vi "RX OOB Test Cases.vi"() -> (0 "error out":errorcluster, 2 "status":string, 3 "pass":bool)   [LabVIEW 2021]
uses:
  CIFUtilities/CIFOutOfBand/CIFOutOfBand.lvclass/CIFOutOfBand.ctl
  OOB_Rx/Typedef/OOB Core Commands.ctl
  OOB_Rx/Private/Command Settings.vi
  CIFUtilities/CIFOutOfBand/Accessors/Write Local OOB Data.vi
  CIFUtilities/CIFOutOfBand/Write OOB DVR.vi
  CIFUtilities/CIFOutOfBand/Utilities/Command to Bitwise Command.vi
  CIFUtilities/CIFOutOfBand/Read OOB DVR.vi
  OOB_Rx/Private/Read Payload.vi
  OOB_Rx/CIFCoreOOB_Rx.lvclass
  D:/dev/CIF-LVCore/src/CIFUtilities/CIFOutOfBand/CIFOutOfBand.lvclass
  CIFUtilities/CIFOutOfBand/Init OOB.vi
  <vilib>/addons/_JKI.lib/Serialization/JSON/Library/Unflatten From JSON String.vi
  <vilib>/addons/_JKI.lib/Serialization/JSON/JKI JSON Serialization.lvlib
  CIFUtilities/CIFOutOfBand/CIFOutOfBand.lvclass
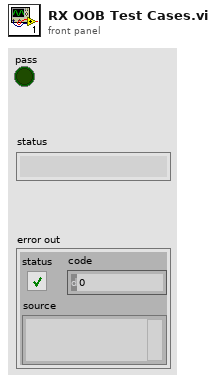
[diagram p1: front panel]
types:
  T1 = cluster{"Numeric":dbl, "Array":cluster{"Numeric":dbl, "String":string, "Boolean":bool}[], "string":string, "Null array":u8[]}
  T2 = typedef "CIFCoreOOB_Rx.lvclass/OOB Core Commands.ctl" = enum8{"Start", "StartFTE", "Pause", "Stop", "RefreshStats", "UpdateConfig"}
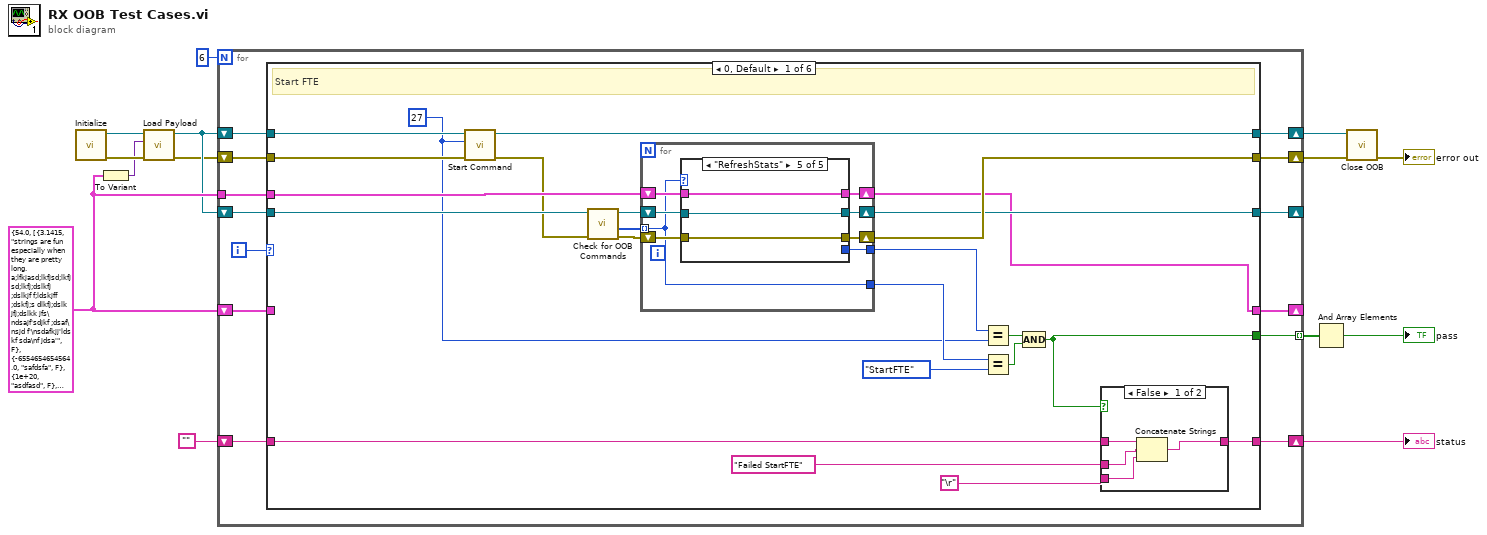
[diagram p0: block diagram]
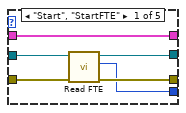
[diagram p2: hidden frame]
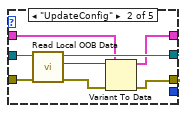
[diagram p3: hidden frame]
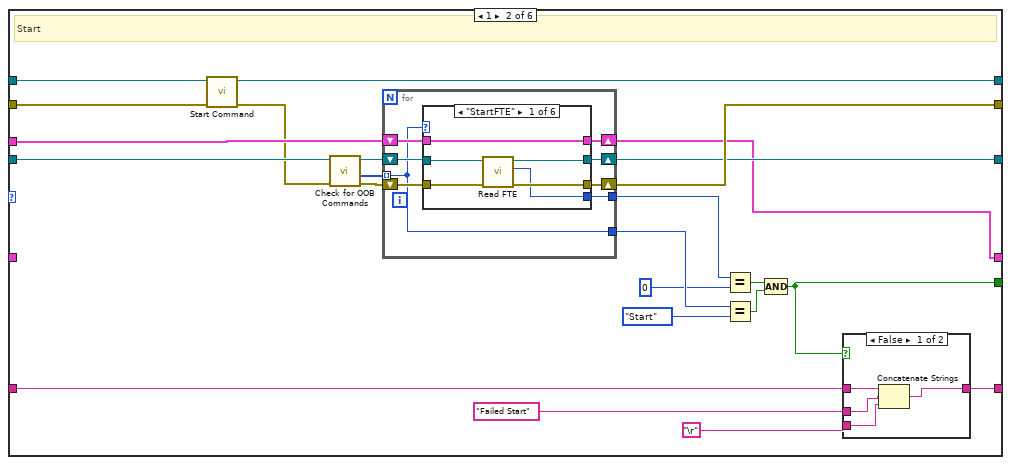
[diagram p7: hidden frame]
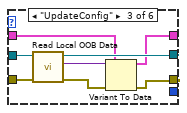
[diagram p9: hidden frame]
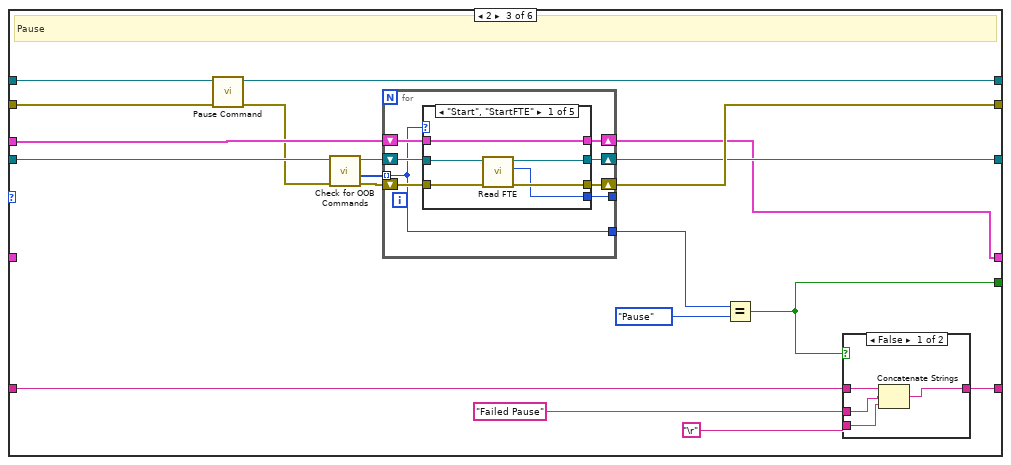
[diagram p14: hidden frame]
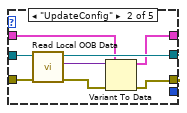
[diagram p15: hidden frame]
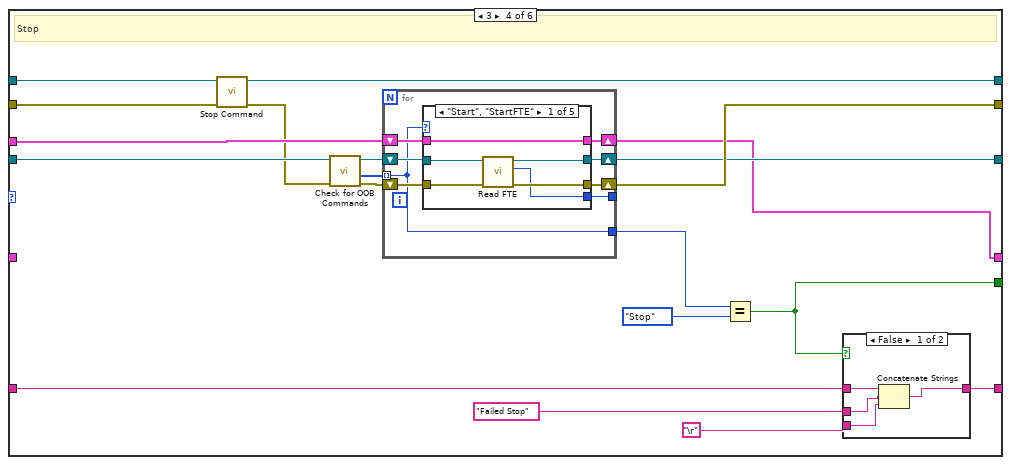
[diagram p20: hidden frame]
diagram:
  w14 = T1 {"Numeric"=54.0, "Array"=[{"Numeric"=3.1415, "String"="strings are fun especially when they are pretty long. a;lfkjasd;lkfjsd;lkfjsd;lkfj;dslkfj ;dslkjf f;ldskjff ;dskfj;s dlkfj;dslk jfj;dslkk jfs\ndsajf'sdjkf ;dsaf\nsjd f'\nsdafkjj'lds kf sda\nf jdsa'", "Boolean"=FALSE}, {"Numeric"=-6554654654564.0, "String"="safdsfa", "Boolean"=FALSE}, {"Numeric"=1e+20, "String"="asdfasd", "Boolean"=FALSE}, {"Numeric"=2.0, "String"="afd", "Boolean"=TRUE}, {"Numeric"=12.34, "String"="data", "Boolean"=FALSE}], "string"="strings", "Null array"=[0]} ("Test Config")
  n1 = call "Initialize.vi"() -> ("error out"=w7:errorcluster, "CoreOOB_Rx out"=w6:refnum<class "CIFCoreOOB_Rx.lvclass">)  [unwired: 10 in]
  n2 = To Variant(anything=w14) -> (Variant=w3:variant)
  n3 = call "Load Payload.vi"("error in (no error)"=w7, "Configuration Payload"=w3, "CoreOOB_Rx in"=w6) -> ("error out"=w4:errorcluster, "CoreOOB_Rx out"=w5:refnum<class "CIFCoreOOB_Rx.lvclass">)  [unwired: 7 in]
  n4 = for {
    N: 6 -> [_]
    tunnel: [w27] -> w11 mode=indexing
    tunnel: w14 -> [w25]
    shift-right: [w23] -> w12
    shift-left: w4 -> [w26]
    shift-right: [w21] -> w13
    shift-left: w5 -> [w24]
    shift-right: [w19] -> _
    shift-left: w5 -> [w20]
    shift-right: [w18] -> _
    shift-left: w14 -> [w17]
    shift-right: [w15] -> w8
    shift-left: "" -> [w16]
    i -> [w22]
    n5 = case shown="0, Default" w22 {
      tunnel: [w32 w91 w149 w208 w263 w325] -> w27
      tunnel: w26 -> [w41 w100 w152 w206 w261 w320]
      tunnel: w25 -> [w50 w109 w167 w222 w277 w318]
      tunnel: w24 -> [w42 w101 w153 w207 w262 w322]
      tunnel: [w49 w108 w166 w221 w276 w337] -> w23
      tunnel: [w40 w99 w150 w204 w259 w321] -> w21
      tunnel: w20 -> [w39 w98 w159 w214 w269 w331]
      tunnel: [w48 w107 w165 w220 w275 w336] -> w19
      tunnel: [w47 w106 w164 w219 w274 w314] -> w18
      tunnel: w17 -> [_ _ _ _ _ _]
      tunnel: w16 -> [w46 w105 w163 w218 w273 w335]
      tunnel: [w45 w104 w162 w217 w272 w334] -> w15
      frame 0, Default {
        w28 = u64 27 ("FTE")
        # "Start FTE"
        n6 = call "Start Command.vi"("error in"=w41, "FTE"=w28, "CoreOOB_Rx in"=w42) -> ("error out"=w38:errorcluster, "CoreOOB_Rx out"=w40:refnum<class "CIFCoreOOB_Rx.lvclass">)  [unwired: 7 in]
        n7 = call "Check for OOB Commands.vi"("error in (no error)"=w38, "CoreOOB_Rx in"=w39) -> ("error out"=w37:errorcluster, "Commands"=w35:T2[], "CoreOOB_Rx out"=w36:refnum<class "CIFCoreOOB_Rx.lvclass">)  [unwired: 6 in, 1 out]
        n8 = for {
          tunnel: w35 -> [w51] mode=indexing
          shift-right: [w53] -> w47
          shift-left: w50 -> [w58]
          shift-right: [w57] -> w49
          shift-left: w37 -> [w55]
          shift-right: [w56] -> w48
          shift-left: w36 -> [w54]
          tunnel: [w52] -> w31
          tunnel: [w51] -> w30
          n9 = case shown="\"RefreshStats\"" w51 {
            tunnel: w54 -> [w64 w72 w74 w77 w80]
            tunnel: w55 -> [w63 w71 w73 w76 w81]
            tunnel: [w62 w69 w74 w77 w80] -> w56
            tunnel: w58 -> [w59 w67 w75 w78 w79]
            tunnel: [w61 w66 w73 w76 w81] -> w57
            tunnel: [w59 w65 w75 w78 w79] -> w53
            tunnel: [w60 _ _ _ _] -> w52
            frame "Start", "StartFTE" {
              n10 = call "Read FTE.vi"("error in"=w63, "CoreOOB_Rx in"=w64) -> ("error out"=w61:errorcluster, "FTE"=w60:u64, "CoreOOB_Rx out"=w62:refnum<class "CIFCoreOOB_Rx.lvclass">)  [unwired: 7 in]
            }
            frame "UpdateConfig" {
              n11 = call "Read Local OOB Data.vi"("error in"=w71, "OOB in"=w72) -> ("error out"=w70:errorcluster, "Local OOB Data"=w68:variant, "OOB out"=w69:refnum<class "CIFCoreOOB_Rx.lvclass">)  [unwired: 7 in]
              n12 = Variant To Data(error in=w70, type=w67, Variant=w68) -> (data=w65:T1, error out=w66:errorcluster)
            }
            frame "Pause" {
            }
            frame "Stop" {
            }
            frame "RefreshStats" {
            }
          }
        }
        n13 = Equal?(x=w31, y=w28) -> (x = y?=w34:bool)
        n14 = Equal?(x=w30, y=OOB_Core_Commands."StartFTE") -> (x = y?=w33:bool)
        n15 = Compound Arithmetic op=AND(w34, w33) -> (w32:bool)
        n16 = case shown="False" w32 {
          tunnel: w46 -> [w85 w86]
          tunnel: [w82 w86] -> w45
          tunnel: "Failed StartFTE" -> [w84 _]
          tunnel: "\r" -> [w83 _]
          frame False {
            n17 = Concatenate Strings(w85, w84, w83) -> (w82:string)
          }
          frame True {
          }
        }
      }
      frame 1 {
        # "Start"
        n18 = call "Start Command.vi"("error in"=w100, "CoreOOB_Rx in"=w101) -> ("error out"=w97:errorcluster, "CoreOOB_Rx out"=w99:refnum<class "CIFCoreOOB_Rx.lvclass">)  [unwired: 8 in]
        n19 = call "Check for OOB Commands.vi"("error in (no error)"=w97, "CoreOOB_Rx in"=w98) -> ("error out"=w96:errorcluster, "Commands"=w94:T2[], "CoreOOB_Rx out"=w95:refnum<class "CIFCoreOOB_Rx.lvclass">)  [unwired: 6 in, 1 out]
        n20 = for {
          tunnel: w94 -> [w110] mode=indexing
          shift-right: [w112] -> w106
          shift-left: w109 -> [w117]
          shift-right: [w116] -> w108
          shift-left: w96 -> [w114]
          shift-right: [w115] -> w107
          shift-left: w95 -> [w113]
          tunnel: [w111] -> w90
          tunnel: [w110] -> w89
          n21 = case shown="\"StartFTE\"" w110 {
            tunnel: w113 -> [w123 w124 w134 w136 w139 w142]
            tunnel: w114 -> [w122 w125 w133 w135 w138 w143]
            tunnel: [w121 w124 w131 w136 w139 w142] -> w115
            tunnel: w117 -> [w118 w126 w129 w137 w140 w141]
            tunnel: [w120 w125 w128 w135 w138 w143] -> w116
            tunnel: [w118 w126 w127 w137 w140 w141] -> w112
            tunnel: [w119 _ _ _ _ _] -> w111
            frame "StartFTE" {
              n22 = call "Read FTE.vi"("error in"=w122, "CoreOOB_Rx in"=w123) -> ("error out"=w120:errorcluster, "FTE"=w119:u64, "CoreOOB_Rx out"=w121:refnum<class "CIFCoreOOB_Rx.lvclass">)  [unwired: 7 in]
            }
            frame "Start" {
            }
            frame "UpdateConfig" {
              n23 = call "Read Local OOB Data.vi"("error in"=w133, "OOB in"=w134) -> ("error out"=w132:errorcluster, "Local OOB Data"=w130:variant, "OOB out"=w131:refnum<class "CIFCoreOOB_Rx.lvclass">)  [unwired: 7 in]
              n24 = Variant To Data(error in=w132, type=w129, Variant=w130) -> (data=w127:T1, error out=w128:errorcluster)
            }
            frame "Pause" {
            }
            frame "Stop" {
            }
            frame "RefreshStats" {
            }
          }
        }
        n25 = Equal?(x=w90, y=u64 0 ("FTE")) -> (x = y?=w93:bool)
        n26 = Equal?(x=w89, y=OOB_Core_Commands."Start") -> (x = y?=w92:bool)
        n27 = Compound Arithmetic op=AND(w93, w92) -> (w91:bool)
        n28 = case shown="False" w91 {
          tunnel: w105 -> [w147 w148]
          tunnel: [w144 w148] -> w104
          tunnel: "Failed Start" -> [w146 _]
          tunnel: "\r" -> [w145 _]
          frame False {
            n29 = Concatenate Strings(w147, w146, w145) -> (w144:string)
          }
          frame True {
          }
        }
      }
      frame 2 {
        # "Pause"
        n30 = call "Pause Command.vi"("error in"=w152, "CoreOOB_Rx in"=w153) -> ("error out"=w151:errorcluster, "CoreOOB_Rx out"=w150:refnum<class "CIFCoreOOB_Rx.lvclass">)  [unwired: 8 in]
        n31 = call "Check for OOB Commands.vi"("error in (no error)"=w151, "CoreOOB_Rx in"=w159) -> ("error out"=w158:errorcluster, "Commands"=w156:T2[], "CoreOOB_Rx out"=w157:refnum<class "CIFCoreOOB_Rx.lvclass">)  [unwired: 6 in, 1 out]
        n32 = for {
          tunnel: w156 -> [w168] mode=indexing
          shift-right: [w170] -> w164
          shift-left: w167 -> [w175]
          shift-right: [w174] -> w166
          shift-left: w158 -> [w172]
          shift-right: [w173] -> w165
          shift-left: w157 -> [w171]
          tunnel: [w169] -> _
          tunnel: [w168] -> w155
          n33 = case shown="\"Start\", \"StartFTE\"" w168 {
            tunnel: w171 -> [w181 w189 w191 w194 w197]
            tunnel: w172 -> [w180 w188 w190 w193 w198]
            tunnel: [w179 w186 w191 w194 w197] -> w173
            tunnel: w175 -> [w176 w184 w192 w195 w196]
            tunnel: [w178 w183 w190 w193 w198] -> w174
            tunnel: [w176 w182 w192 w195 w196] -> w170
            tunnel: [w177 _ _ _ _] -> w169
            frame "Start", "StartFTE" {
              n34 = call "Read FTE.vi"("error in"=w180, "CoreOOB_Rx in"=w181) -> ("error out"=w178:errorcluster, "FTE"=w177:u64, "CoreOOB_Rx out"=w179:refnum<class "CIFCoreOOB_Rx.lvclass">)  [unwired: 7 in]
            }
            frame "UpdateConfig" {
              n35 = call "Read Local OOB Data.vi"("error in"=w188, "OOB in"=w189) -> ("error out"=w187:errorcluster, "Local OOB Data"=w185:variant, "OOB out"=w186:refnum<class "CIFCoreOOB_Rx.lvclass">)  [unwired: 7 in]
              n36 = Variant To Data(error in=w187, type=w184, Variant=w185) -> (data=w182:T1, error out=w183:errorcluster)
            }
            frame "Pause" {
            }
            frame "Stop" {
            }
            frame "RefreshStats" {
            }
          }
        }
        n37 = Equal?(x=w155, y=OOB_Core_Commands."Pause") -> (x = y?=w149:bool)
        n38 = case shown="False" w149 {
          tunnel: w163 -> [w202 w203]
          tunnel: [w199 w203] -> w162
          tunnel: "Failed Pause" -> [w201 _]
          tunnel: "\r" -> [w200 _]
          frame False {
            n39 = Concatenate Strings(w202, w201, w200) -> (w199:string)
          }
          frame True {
          }
        }
      }
      frame 3 {
        # "Stop"
        n40 = call "Stop Command.vi"("error in"=w206, "CoreOOB_Rx in"=w207) -> ("error out"=w205:errorcluster, "CoreOOB_Rx out"=w204:refnum<class "CIFCoreOOB_Rx.lvclass">)  [unwired: 8 in]
        n41 = call "Check for OOB Commands.vi"("error in (no error)"=w205, "CoreOOB_Rx in"=w214) -> ("error out"=w213:errorcluster, "Commands"=w211:T2[], "CoreOOB_Rx out"=w212:refnum<class "CIFCoreOOB_Rx.lvclass">)  [unwired: 6 in, 1 out]
        n42 = for {
          tunnel: w211 -> [w223] mode=indexing
          shift-right: [w225] -> w219
          shift-left: w222 -> [w230]
          shift-right: [w229] -> w221
          shift-left: w213 -> [w227]
          shift-right: [w228] -> w220
          shift-left: w212 -> [w226]
          tunnel: [w224] -> _
          tunnel: [w223] -> w210
          n43 = case shown="\"Start\", \"StartFTE\"" w223 {
            tunnel: w226 -> [w236 w244 w246 w249 w252]
            tunnel: w227 -> [w235 w243 w245 w248 w253]
            tunnel: [w234 w241 w246 w249 w252] -> w228
            tunnel: w230 -> [w231 w239 w247 w250 w251]
            tunnel: [w233 w238 w245 w248 w253] -> w229
            tunnel: [w231 w237 w247 w250 w251] -> w225
            tunnel: [w232 _ _ _ _] -> w224
            frame "Start", "StartFTE" {
              n44 = call "Read FTE.vi"("error in"=w235, "CoreOOB_Rx in"=w236) -> ("error out"=w233:errorcluster, "FTE"=w232:u64, "CoreOOB_Rx out"=w234:refnum<class "CIFCoreOOB_Rx.lvclass">)  [unwired: 7 in]
            }
            frame "UpdateConfig" {
              n45 = call "Read Local OOB Data.vi"("error in"=w243, "OOB in"=w244) -> ("error out"=w242:errorcluster, "Local OOB Data"=w240:variant, "OOB out"=w241:refnum<class "CIFCoreOOB_Rx.lvclass">)  [unwired: 7 in]
              n46 = Variant To Data(error in=w242, type=w239, Variant=w240) -> (data=w237:T1, error out=w238:errorcluster)
            }
            frame "Pause" {
            }
            frame "Stop" {
            }
            frame "RefreshStats" {
            }
          }
        }
        n47 = Equal?(x=w210, y=OOB_Core_Commands."Stop") -> (x = y?=w208:bool)
        n48 = case shown="False" w208 {
          tunnel: w218 -> [w257 w258]
          tunnel: [w254 w258] -> w217
          tunnel: "Failed Stop" -> [w256 _]
          tunnel: "\r" -> [w255 _]
          frame False {
            n49 = Concatenate Strings(w257, w256, w255) -> (w254:string)
          }
          frame True {
          }
        }
      }
      frame 4 {
        # "Refresh"
        n50 = call "Refresh Stats Command.vi"("error in"=w261, "CoreOOB_Rx in"=w262) -> ("error out"=w260:errorcluster, "CoreOOB_Rx out"=w259:refnum<class "CIFCoreOOB_Rx.lvclass">)  [unwired: 8 in]
        n51 = call "Check for OOB Commands.vi"("error in (no error)"=w260, "CoreOOB_Rx in"=w269) -> ("error out"=w268:errorcluster, "Commands"=w266:T2[], "CoreOOB_Rx out"=w267:refnum<class "CIFCoreOOB_Rx.lvclass">)  [unwired: 6 in, 1 out]
        n52 = for {
          tunnel: w266 -> [w278] mode=indexing
          shift-right: [w280] -> w274
          shift-left: w277 -> [w285]
          shift-right: [w284] -> w276
          shift-left: w268 -> [w282]
          shift-right: [w283] -> w275
          shift-left: w267 -> [w281]
          tunnel: [w279] -> _
          tunnel: [w278] -> w265
          n53 = case shown="\"RefreshStats\"" w278 {
            tunnel: w281 -> [w291 w299 w301 w304 w307]
            tunnel: w282 -> [w290 w298 w300 w303 w308]
            tunnel: [w289 w296 w301 w304 w307] -> w283
            tunnel: w285 -> [w286 w294 w302 w305 w306]
            tunnel: [w288 w293 w300 w303 w308] -> w284
            tunnel: [w286 w292 w302 w305 w306] -> w280
            tunnel: [w287 _ _ _ _] -> w279
            frame "Start", "StartFTE" {
              n54 = call "Read FTE.vi"("error in"=w290, "CoreOOB_Rx in"=w291) -> ("error out"=w288:errorcluster, "FTE"=w287:u64, "CoreOOB_Rx out"=w289:refnum<class "CIFCoreOOB_Rx.lvclass">)  [unwired: 7 in]
            }
            frame "UpdateConfig" {
              n55 = call "Read Local OOB Data.vi"("error in"=w298, "OOB in"=w299) -> ("error out"=w297:errorcluster, "Local OOB Data"=w295:variant, "OOB out"=w296:refnum<class "CIFCoreOOB_Rx.lvclass">)  [unwired: 7 in]
              n56 = Variant To Data(error in=w297, type=w294, Variant=w295) -> (data=w292:T1, error out=w293:errorcluster)
            }
            frame "Pause" {
            }
            frame "Stop" {
            }
            frame "RefreshStats" {
            }
          }
        }
        n57 = Equal?(x=w265, y=OOB_Core_Commands."RefreshStats") -> (x = y?=w263:bool)
        n58 = case shown="False" w263 {
          tunnel: w273 -> [w312 w313]
          tunnel: [w309 w313] -> w272
          tunnel: "Failed Refresh" -> [w311 _]
          tunnel: "\r" -> [w310 _]
          frame False {
            n59 = Concatenate Strings(w312, w311, w310) -> (w309:string)
          }
          frame True {
          }
        }
      }
      frame 5 {
        # "Update Config"
        n60 = Bundle By Name(cluster=w318, "Numeric"=86.0) -> (w315:T1)
        n61 = call <vilib>:"Flatten To JSON String.vi"("Variant"=w315) -> ("JSON String"=w316:string)  [unwired: 9 in, 1 out]
        n62 = call "Update Configuration Command.vi"("error in"=w320, "Config JSON"=w316, "CoreOOB_Rx in"=w322) -> ("error out"=w319:errorcluster, "CoreOOB_Rx out"=w321:refnum<class "CIFCoreOOB_Rx.lvclass">)  [unwired: 7 in]
        n63 = call "Check for OOB Commands.vi"("error in (no error)"=w319, "CoreOOB_Rx in"=w331) -> ("error out"=w330:errorcluster, "Commands"=w328:T2[], "CoreOOB_Rx out"=w329:refnum<class "CIFCoreOOB_Rx.lvclass">)  [unwired: 6 in, 1 out]
        n64 = for {
          tunnel: w328 -> [w338] mode=indexing
          shift-right: [w340] -> w314
          shift-left: w318 -> [w345]
          shift-right: [w344] -> w337
          shift-left: w330 -> [w342]
          shift-right: [w343] -> w336
          shift-left: w329 -> [w341]
          tunnel: [w339] -> _
          tunnel: [w338] -> w324
          n65 = case shown="\"UpdateConfig\"" w338 {
            tunnel: w341 -> [w351 w355 w361 w364 w367]
            tunnel: w342 -> [w350 w356 w360 w363 w368]
            tunnel: [w349 w354 w361 w364 w367] -> w343
            tunnel: w345 -> [w346 w359 w362 w365 w366]
            tunnel: [w348 w358 w360 w363 w368] -> w344
            tunnel: [w346 w357 w362 w365 w366] -> w340
            tunnel: [w347 _ _ _ _] -> w339
            frame "Start", "StartFTE" {
              n66 = call "Read FTE.vi"("error in"=w350, "CoreOOB_Rx in"=w351) -> ("error out"=w348:errorcluster, "FTE"=w347:u64, "CoreOOB_Rx out"=w349:refnum<class "CIFCoreOOB_Rx.lvclass">)  [unwired: 7 in]
            }
            frame "UpdateConfig" {
              n67 = call "Read Configuration.vi"("error in"=w356, "CoreOOB_Rx in"=w355) -> ("error out"=w352:errorcluster, "Configuration Data"=w353:variant, "CoreOOB_Rx out"=w354:refnum<class "CIFCoreOOB_Rx.lvclass">)  [unwired: 7 in]
              n68 = Variant To Data(error in=w352, type=w359, Variant=w353) -> (data=w357:T1, error out=w358:errorcluster)
            }
            frame "Pause" {
            }
            frame "Stop" {
            }
            frame "RefreshStats" {
            }
          }
        }
        n69 = Equal?(x=w314, y=w315) -> (x = y?=w327:bool)
        n70 = Equal?(x=w324, y=OOB_Core_Commands."UpdateConfig") -> (x = y?=w326:bool)
        n71 = Compound Arithmetic op=AND(w327, w326) -> (w325:bool)
        n72 = case shown="False" w325 {
          tunnel: w335 -> [w372 w373]
          tunnel: [w369 w373] -> w334
          tunnel: "Failed Update Config" -> [w371 _]
          tunnel: "\r" -> [w370 _]
          frame False {
            n73 = Concatenate Strings(w372, w371, w370) -> (w369:string)
          }
          frame True {
          }
        }
      }
    }
  }
  "status" <- w8
  n74 = And Array Elements(Boolean array=w11) -> (logical AND=→"pass":bool)
  n75 = call "Close OOB.vi"("error in"=w12, "OOB in"=w13) -> ("error out"=→"error out":errorcluster)  [unwired: 9 in]
